vi "STRING_POT_CAL 2016.vi"(6 "Sensor Cluster":T1, 7 "Array in":refnum<k24>[](array[refnum]), 8 "error in (no error)":errorcluster, 9 "Descriptions":string[](array[string]), 11 "string_pot_slope_IN":dbl=51.35 format="%.2f") -> (0 "error out":errorcluster, 3 "string_pot_slope_OUT":dbl=51.35 format="%.2f", 4 "Sensor Cluster 2":T1, 5 "Array out":refnum<k24>[](array[refnum]))   [LabVIEW 2016]
uses:
  C:/Program Files (x86)/National Instruments/LabVIEW 2016/vi.lib/ULx/ULx_LV.dll
  Waterloo DAQ/controls/MCC DAQ Readings.ctl
  KPRO_lv2015/ad interface/Global_SIM_switch.vi
  KPRO_lv2015/Kpro Globals.vi
panel:
  in  "Calibration \nDistance":dbl=5.0 format="%#_13g"
  out "String Pot \nSlope":dbl=1.7339999675750732 format="%.2f"
  out "delta Distance":dbl
  out "Distance(ft)":dbl format="%.2f"
  in  "stop":bool
  in  "start":bool
  # "STRING POTENTIOMETER CALIBRATION"
  # "Hold string pot wire at 5' above the string pot body.\nPress start."
  # "Slowly lower the string pot wire.\nPress Stop when t he string pot wire is fully retracted."
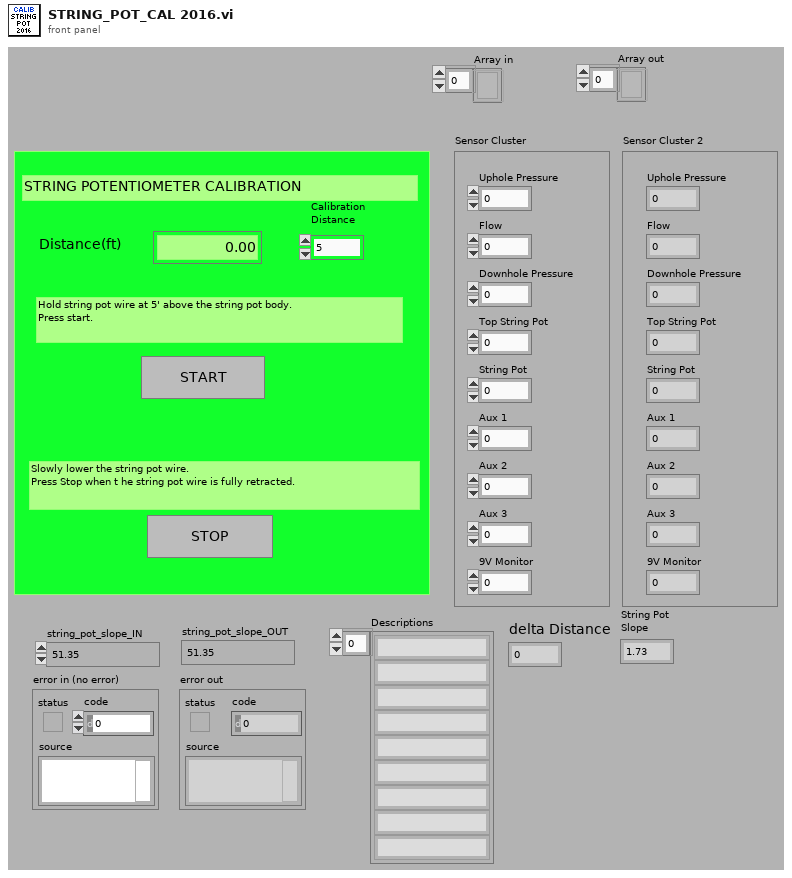
[diagram p1: front panel]
types:
  T1 = typedef "MCC DAQ Readings.ctl" = cluster{"Uphole Pressure":dbl, "Flow":dbl, "Downhole Pressure":dbl, "Top String Pot":dbl, "String Pot":dbl, "Aux 1":dbl, "Aux 2":dbl, "Aux 3":dbl, "9V Monitor":dbl}
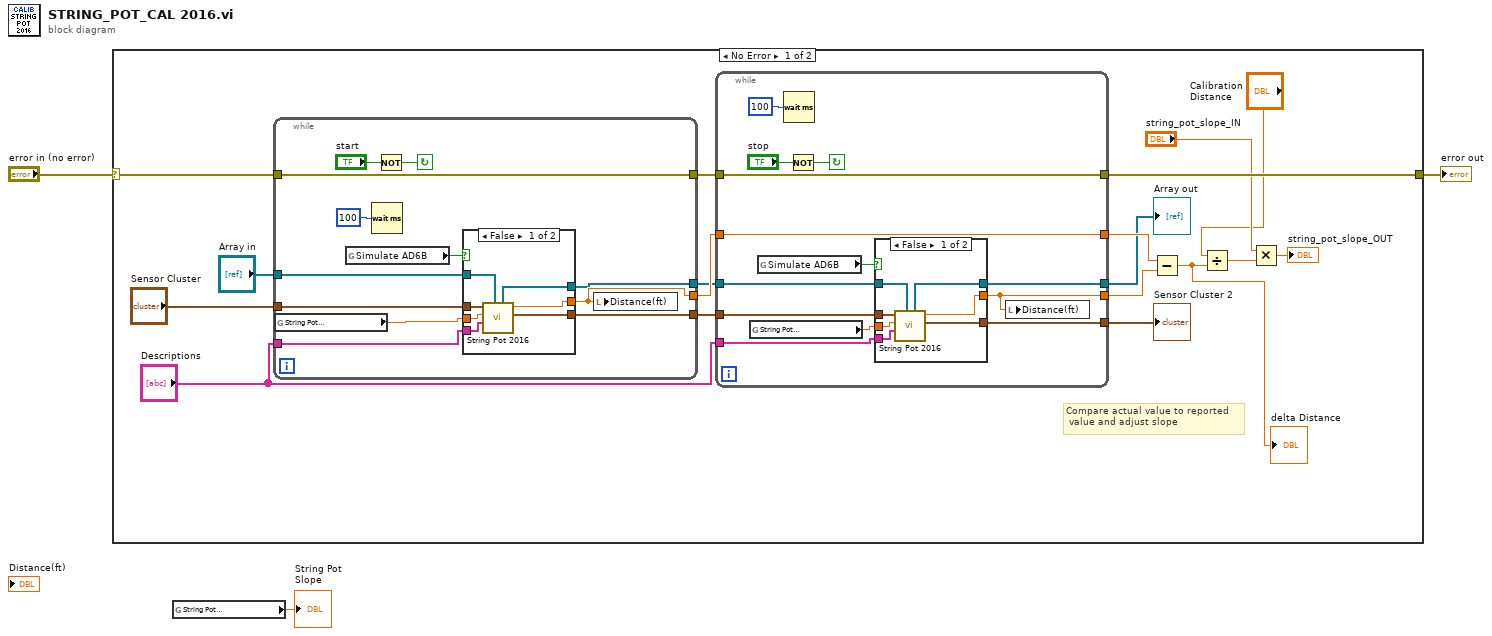
[diagram p0: block diagram]
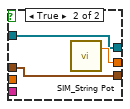
[diagram p2: hidden frame]
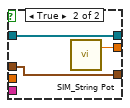
[diagram p3: hidden frame]
diagram:
  n1 = case shown="No Error" "error in (no error)" {
    selector: "error in (no error)" -> [w21 w67]
    tunnel: [w19 w67] -> w3
    frame No Error {
      # "Compare actual value to reported\n value and adjust slope"
      n2 = while {
        tunnel: [w28] -> w16
        tunnel: [w31] -> w20
        tunnel: w21 -> [w31]
        tunnel: "Array in" -> [w27]
        tunnel: "Sensor Cluster" -> [w26]
        tunnel: "Descriptions" -> [w25]
        tunnel: [w24] -> w7
        tunnel: [w23] -> w9
        stop <- w32 continue-if-true
        n3 = global read "Kpro Globals.vi" "String Pot \nSlope"() -> (w22:dbl)
        n4 = global read "Global_SIM_switch.vi" "Simulate AD6B"() -> (w30:bool)
        n5 = Wait (ms)(milliseconds to wait=u32 100) -> ()  [unwired: 1 out]
        n6 = Not(x="start") -> (.not. x?=w32:bool)
        n7 = case shown="False" w30 {
          tunnel: [w40 w43] -> w28
          tunnel: w27 -> [w39 w41]
          tunnel: w26 -> [w38 w42]
          tunnel: w25 -> [w37 _]
          tunnel: [w36 w42] -> w24
          tunnel: [w35 w41] -> w23
          tunnel: w22 -> [w34 _]
          frame False {
            n8 = call "String Pot 2016.vi"("Array in"=w39, "Descriptions"=w37, "String Pot \nSlope"=w34, "Sensor Cluster"=w38) -> ("Sensor Cluster 2"=w36:T1, "Distance (in)"=w40:dbl, "Array out"=w35:refnum<k24>[])  [unwired: 4 in, 1 out]
          }
          frame True {
            n9 = call "SIM_String Pot.vi"() -> ("Distance (in)"=w43:dbl)  [unwired: 3 in]
          }
        }
        n10 = local write "Distance(ft)"(w28) -> ()
      }
      n11 = while {
        tunnel: w16 -> [w53]
        tunnel: [w51] -> w14
        tunnel: [w53] -> w13
        tunnel: w20 -> [w54]
        tunnel: [w54] -> w19
        tunnel: "Descriptions" -> [w49]
        tunnel: w9 -> [w48]
        tunnel: [w47] -> w8
        tunnel: w7 -> [w45]
        tunnel: [w44] -> w6
        stop <- w56 continue-if-true
        n12 = global read "Kpro Globals.vi" "String Pot \nSlope"() -> (w46:dbl)
        n13 = global read "Global_SIM_switch.vi" "Simulate AD6B"() -> (w50:bool)
        n14 = Wait (ms)(milliseconds to wait=u32 100) -> ()  [unwired: 1 out]
        n15 = Not(x="stop") -> (.not. x?=w56:bool)
        n16 = case shown="False" w50 {
          tunnel: [w63 w66] -> w51
          tunnel: w48 -> [w62 w64]
          tunnel: w45 -> [w61 w65]
          tunnel: w49 -> [w60 _]
          tunnel: [w59 w65] -> w44
          tunnel: [w58 w64] -> w47
          tunnel: w46 -> [w57 _]
          frame False {
            n17 = call "String Pot 2016.vi"("Array in"=w62, "Descriptions"=w60, "String Pot \nSlope"=w57, "Sensor Cluster"=w61) -> ("Sensor Cluster 2"=w59:T1, "Distance (in)"=w63:dbl, "Array out"=w58:refnum<k24>[])  [unwired: 4 in, 1 out]
          }
          frame True {
            n18 = call "SIM_String Pot.vi"() -> ("Distance (in)"=w66:dbl)  [unwired: 3 in]
          }
        }
        n19 = local write "Distance(ft)"(w51) -> ()
      }
      "Sensor Cluster 2" <- w6
      "Array out" <- w8
      n20 = Subtract(x=w13, y=w14) -> (x-y=w4:dbl)
      "delta Distance" <- w4
      n21 = Divide(x="Calibration \nDistance", y=w4) -> (x/y=w15:dbl)
      n22 = Multiply(x="string_pot_slope_IN", y=w15) -> (x*y=→"string_pot_slope_OUT":dbl)
    }
    frame Error {
    }
  }
  "error out" <- w3
  n23 = global read "Kpro Globals.vi" "String Pot \nSlope"() -> (→"String Pot \nSlope":dbl)
